vi "Fill DataTable.vi"   [LabVIEW 2019, in "JMP Automation.lvlib"]
doc: "Add columns with their coresponding data to a DataDable"
uses:
  <instrlib>/LV_JMP_bridge/JMP Automation.lvlib
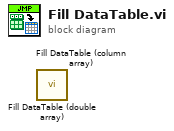
[diagram p0: block diagram]
diagram:
  n1 = call <instrlib>:"Fill DataTable (double array).vi"() -> ()  [unwired: 10 in, 2 out]
  n2 = call <instrlib>:"Fill DataTable (column array).vi"() -> ()  [unwired: 10 in, 2 out]
